vi "get_path_sfx.vi"(8 "error in (no error)":errorcluster) -> (0 "error out":errorcluster, 3 "sfx":path)   [LabVIEW 2015, in "lv-bin-7zip.lvlib"]
uses:
  lv-bin-7zip.lvlib
  public/_controls/error.ctl
  <userlib>/antonio-alexander/lv-bin/public/api/v1/v1.lvlib
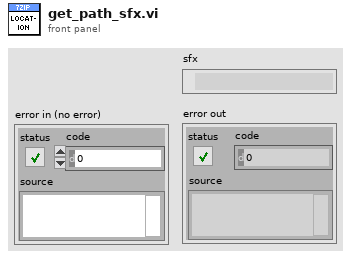
[diagram p1: front panel]
types:
  T1 = typedef "lv-bin-7zip.lvlib/error.ctl" = enum16{"null", "exe_x86_missing", "exe_x64_missing", "7za_x86_missing", "7za_x64_missing", "7zxa_x86_missing", "7zxa_x64_missing", "7zS.sfx_missing"}
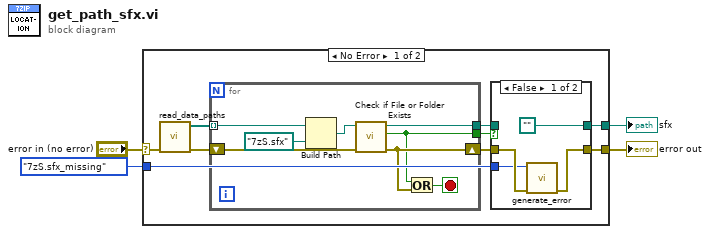
[diagram p0: block diagram]
diagram:
  n1 = case shown="No Error" "error in (no error)" {
    selector: "error in (no error)" -> [w13 w28]
    tunnel: [w6 w28] -> w3
    tunnel: [w8 _] -> w4
    tunnel: error."7zS.sfx_missing" ("error") -> [w5 _]
    frame No Error {
      n2 = call <userlib>:"read_data_paths.vi"("error in (no error)"=w13) -> ("error out"=w12:errorcluster, "path [] out"=w11:path[])  [unwired: 9 in]
      n3 = for {
        tunnel: w11 -> [w19] mode=indexing
        shift-right: [w18] -> w7
        shift-left: w12 -> [w21]
        tunnel: [w20] -> w10
        tunnel: [w16] -> w9
        stop <- w17 stop-if-true
        n4 = Build Path(base path=w19, name or relative path=path "7zS.sfx" ("Application Directory")) -> (appended path=w15:path)
        n5 = call <vilib>:"Check if File or Folder Exists.vi"("error in (no error)"=w21, "path"=w15) -> ("error out"=w18:errorcluster, "file or folder exists?"=w16:bool, "dup path"=w20:path)  [unwired: 7 in]
        n6 = Or(x=w16, y=w18) -> (x .or. y?=w17:bool)
      }
      n7 = case shown="False" w9 {
        tunnel: w10 -> [_ w27]
        tunnel: [path "" w27] -> w8
        tunnel: w7 -> [w25 w26]
        tunnel: [w24 w26] -> w6
        tunnel: w5 -> [w22 _]
        frame False {
          n8 = call "generate_error.vi"("error in (no error)"=w25, "error"=w22) -> ("error out"=w24:errorcluster)  [unwired: 9 in]
        }
        frame True {
        }
      }
    }
    frame Error {
    }
  }
  "error out" <- w3
  "sfx" <- w4
